vi "Blinking LED.vi"() -> ()   [LabVIEW 2017]
uses:
  IMAQCV/GPIO/GPIO Pins.ctl
  <vilib>/Platform/TimedLoop/XDataNode/timing_clust.ctl
  <vilib>/Platform/TimedLoop/XDataNode/nitl_modes.ctl
  <vilib>/Platform/TimedLoop/XDataNode/wakeup.ctl
  <vilib>/platform/TimedLoop/XDataNode/XDataNode.xnode
  <vilib>/Platform/TimedLoop/XDataNode/XDNodeRunTimeDep.lvlib
  IMAQCV/PIIO.lvlib
panel:
  in  "GPIO":T1=41 items=["DI-CH1"=34, "DI-CH2"=35, "DI-CH3"=36, "DI-CH4"=37, "DO-CH1"=41, "DO-CH2"=40, "DO-CH3"=39, "DO-CH4"=38]
  in  "stop":bool
  out "LED1":bool
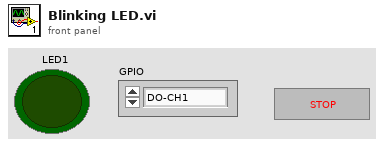
[diagram p1: front panel]
types:
  T1 = typedef "PIIO.lvlib/GPIO Pins.ctl" = u8
  T2 = enum8{"INPUT", "OUTPUT", "PWM_OUTPUT", "GPIO_CLOCK", "SOFT_PWM_OUTPUT", "SOFT_TONE_OUTPUT", "PWM_TONE_OUTPUT"}
  T3 = typedef "XDNodeRunTimeDep.lvlib/timing_clust.ctl" = cluster{"Expected End [f-1]":u64, "Actual End [f-1]":u64, "Finished Late? [f-1]":bool, "Expected End [i-1]":u64, "Actual End [i-1]":u64, "Finished Late? [i-1]":bool, "Expected Start [i]":u64, "Actual Start [i]":u64, "Expected Start [f]":u64, "Actual Start [f]":u64, "Source Name":string, "Structure Name":string, "Period":i64, "Deadline":i64, "Offset":i64, "Start":i64, "Priority":i32, "Timeout":i32, "Mode":T4, "Wakeup Reason":T5, "Error":errorcluster, "Source Type":string, "Secondary Source Type":string, "Global End Time":u64, "Global Start Time":u64, "Frame Duration":u64, "Iteration Duration":u64, "Assigned CPU":i32, "I/O Scan Engine Mode":u32}
  T4 = typedef "XDNodeRunTimeDep.lvlib/nitl_modes.ctl" = enum32{"No Change", "Process missed periods, maintain original phase", "Discard missed periods, maintain original phase", "Process missed periods, ignore original phase", "Discard missed periods, ignore original phase"}
  T5 = typedef "XDNodeRunTimeDep.lvlib/wakeup.ctl" = enum32{"Normal", "Aborted", "Asynchronous wakeup", "Timing source error", "Timed loop error", "Timeout"}
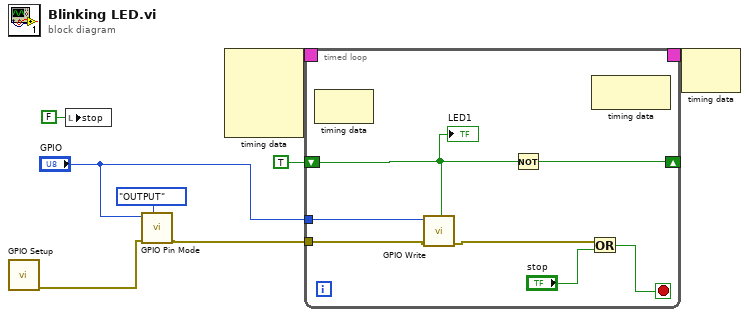
[diagram p0: block diagram]
diagram:
  n1 = call "GPIO Setup.vi"() -> ("error out"=w3:errorcluster)  [unwired: 11 in]
  n2 = local write "stop"(FALSE ("stop")) -> ()
  n3 = call "GPIO Pin Mode.vi"("Pin Mode"=T2."OUTPUT", "error in (no error)"=w3, "GPIO"="GPIO") -> ("error out"=w2:errorcluster)  [unwired: 8 in]
  n4 = node-c288() -> (w6:T3)  [unwired: 4 in]
  n5 = timed-loop {
    tunnel: w2 -> [w10]
    shift-right: [w15] -> _
    shift-left: TRUE -> [w12]
    timing: w6 -> [_]
    timing-out: [_] -> w5
    tunnel: "GPIO" -> [w11]
    stop <- w14 stop-if-true
    n6 = node-c288() -> ()  [unwired: 1 in, 1 out]
    n7 = call "GPIO Write.vi"("Value"=w12, "error in (no error)"=w10, "GPIO"=w11) -> ("error out"=w9:errorcluster)  [unwired: 8 in]
    n8 = Not(x=w12) -> (.not. x?=w15:bool)
    n9 = Or(x=w9, y="stop") -> (x .or. y?=w14:bool)
    n10 = node-c288() -> ()  [unwired: 1 in, 1 out]
    "LED1" <- w12
  }
  n11 = node-c288(w5) -> ()  [unwired: 1 out]
